vi "dfd_SCL_SOSIIRIm_CU.vi"(8 "output valid":bool, 9 "global reset":bool) -> (3 "control state out":T2, 5 "MEM control":T1)   [LabVIEW 2017]
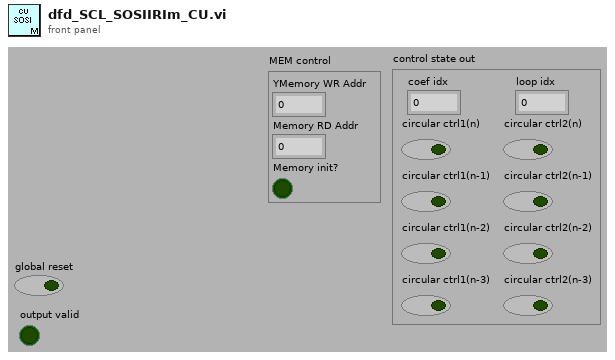
[diagram p1: front panel]
types:
  T1 = cluster{"YMemory WR Addr":u16, "Memory RD Addr":u16, "Memory init?":bool}
  T2 = cluster{"coef idx":u8, "loop idx":u8, "circular ctrl1(n)":bool, "circular ctrl1(n-1)":bool, "circular ctrl1(n-2)":bool, "circular ctrl1(n-3)":bool, "circular ctrl2(n)":bool, "circular ctrl2(n-1)":bool, "circular ctrl2(n-2)":bool, "circular ctrl2(n-3)":bool}
  T3 = cluster{"MEM RD Addr":u16, "Ch cnt":u8, "first run?":bool}
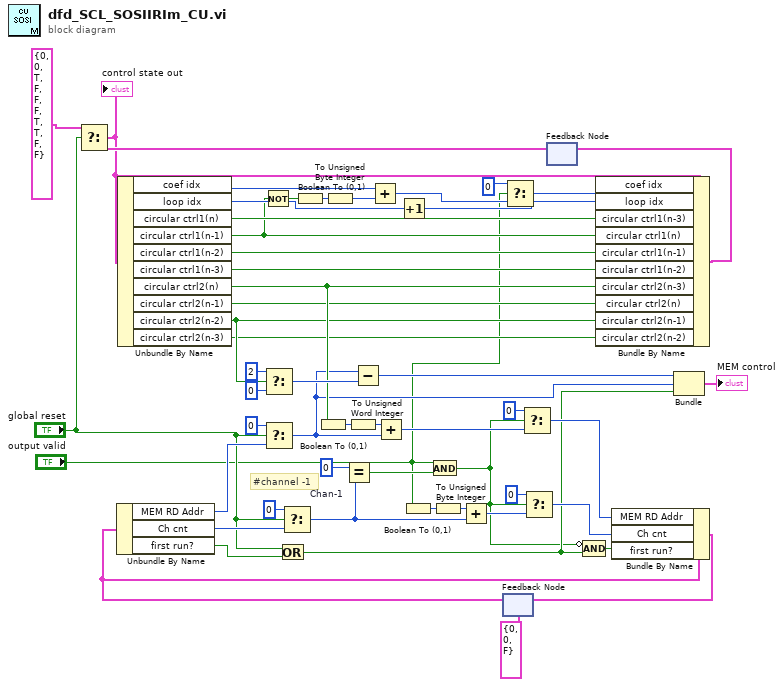
[diagram p0: block diagram]
diagram:
  w43 = u8 0  # Chan-1
  # "#channel -1"
  n1 = Boolean To (0,1)(Boolean="output valid") -> (0, 1=w41:i16)
  n2 = To Unsigned Byte Integer(number=w41) -> (unsigned 8bit integer=w19:u8)
  n3 = feedback #1(T3 {"MEM RD Addr"=0, "Ch cnt"=0, "first run?"=FALSE} ("counter state out")) -> (w12:T3)
  n4 = Unbundle By Name(w12) -> ("MEM RD Addr"=w52:u16, "Ch cnt"=w51:u8, "first run?"=w37:bool)
  n5 = Select(t=u16 0, s="global reset", f=w52) -> (s? t:f=w15:u16)
  n6 = Or(x="global reset", y=w37) -> (x .or. y?=w14:bool)
  n7 = Select(t=u8 0, s="global reset", f=w51) -> (s? t:f=w18:u8)
  n8 = Equal?(x=w43, y=w18) -> (x = y?=w42:bool)
  n9 = And(x="output valid", y=w42) -> (x .and. y?=w5:bool)
  n10 = Add(x=w19, y=w18) -> (x+y=w39:u8)
  n11 = Select(t=u8 0, s=w5, f=w39) -> (s? t:f=w38:u8)
  n12 = feedback #2() -> (w9:T2)  [unwired: 1 out]
  n13 = Select(t=T2 {"coef idx"=0, "loop idx"=0, "circular ctrl1(n)"=TRUE, "circular ctrl1(n-1)"=FALSE, "circular ctrl1(n-2)"=FALSE, "circular ctrl1(n-3)"=FALSE, "circular ctrl2(n)"=TRUE, "circular ctrl2(n-1)"=TRUE, "circular ctrl2(n-2)"=FALSE, "circular ctrl2(n-3)"=FALSE} ("control state in"), s="global reset", f=w9) -> (s? t:f=w6:T2)
  "control state out" <- w6
  n14 = Unbundle By Name(w6) -> ("coef idx"=w45:u8, "loop idx"=w44:u8, "circular ctrl1(n)"=w27:bool, "circular ctrl1(n-1)"=w26:bool, "circular ctrl1(n-2)"=w25:bool, "circular ctrl1(n-3)"=w24:bool, "circular ctrl2(n)"=w23:bool, "circular ctrl2(n-1)"=w22:bool, "circular ctrl2(n-2)"=w21:bool, "circular ctrl2(n-3)"=w20:bool)
  n15 = Not(x=w26) -> (.not. x?=w48:bool)
  n16 = Select(t=u16 2, s=w21, f=u16 0) -> (s? t:f=w28:u16)
  n17 = Boolean To (0,1)(Boolean=w48) -> (0, 1=w47:i16)
  n18 = Boolean To (0,1)(Boolean=w23) -> (0, 1=w35:i16)
  n19 = To Unsigned Byte Integer(number=w47) -> (unsigned 8bit integer=w46:u8)
  n20 = To Unsigned Word Integer(number=w35) -> (unsigned 16bit integer=w34:u16)
  n21 = Subtract(x=w15, y=w28) -> (x-y=w17:u16)
  n22 = Add(x=w45, y=w46) -> (x+y=w2:u8)
  n23 = Add(x=w34, y=w15) -> (x+y=w32:u16)
  n24 = Increment(x=w44) -> (x+1=w49:u8)
  n25 = Select(t=u8 0, s="output valid", f=w2) -> (s? t:f=w3:u8)
  n26 = Select(t=u16 0, s=w5, f=w32) -> (s? t:f=w31:u16)
  n27 = Compound Arithmetic op=AND(invert w5, w14) -> (w36:bool)
  n28 = Bundle By Name(cluster=w6, "coef idx"=w3, "loop idx"=w49, "circular ctrl1(n-3)"=w27, "circular ctrl1(n)"=w26, "circular ctrl1(n-1)"=w25, "circular ctrl1(n-2)"=w24, "circular ctrl2(n-3)"=w23, "circular ctrl2(n)"=w22, "circular ctrl2(n-1)"=w21, "circular ctrl2(n-2)"=w20) -> (w7:T2)
  n29 = feedback-in #2(w7) -> ()
  n30 = Bundle By Name(cluster=w12, "MEM RD Addr"=w31, "Ch cnt"=w38, "first run?"=w36) -> (w13:T3)
  n31 = feedback-in #1(w13) -> ()
  n32 = Bundle(w17, "MEM RD Addr"=w15, w14) -> (→"MEM control":cluster{u16, "MEM RD Addr":u16, bool})  [unwired: 1 out]
